vi "数据查询_数据查询.vi"() -> ()   [LabVIEW 2016, in "数据查询.lvlib"]
uses:
  <vilib>/Utility/miscctls.llb/LVPointTypeDef.ctl
  <userlib>/_LVST/sqlite_api/Core/Select/SQLite_Select Str.vi
  <userlib>/_OpenG.lib/array/array.llb/Sort 2D Array (String)__ogtk.vi
  <vilib>/ptbypt/NI_PtbyPt.lvlib
  System.Windows.Forms
panel:
  in  "数据类型":string(combo)="N"
  out "columns":string[](array[string])
  out "表格":string[][](table)
  in  "是否剔除异常数据":bool=TRUE
  in  "WebBrowser":refnum<k24>(container)
  in  "列表框":i32(listbox)
  in  "导出":bool
  in  "测量模式":string(combo)="全部数据"
  out "选中数据表":string
  in  "查询":bool
  in  "结束日期":string="2050/01/01"
  in  "起始日期":string="2010/01/01"
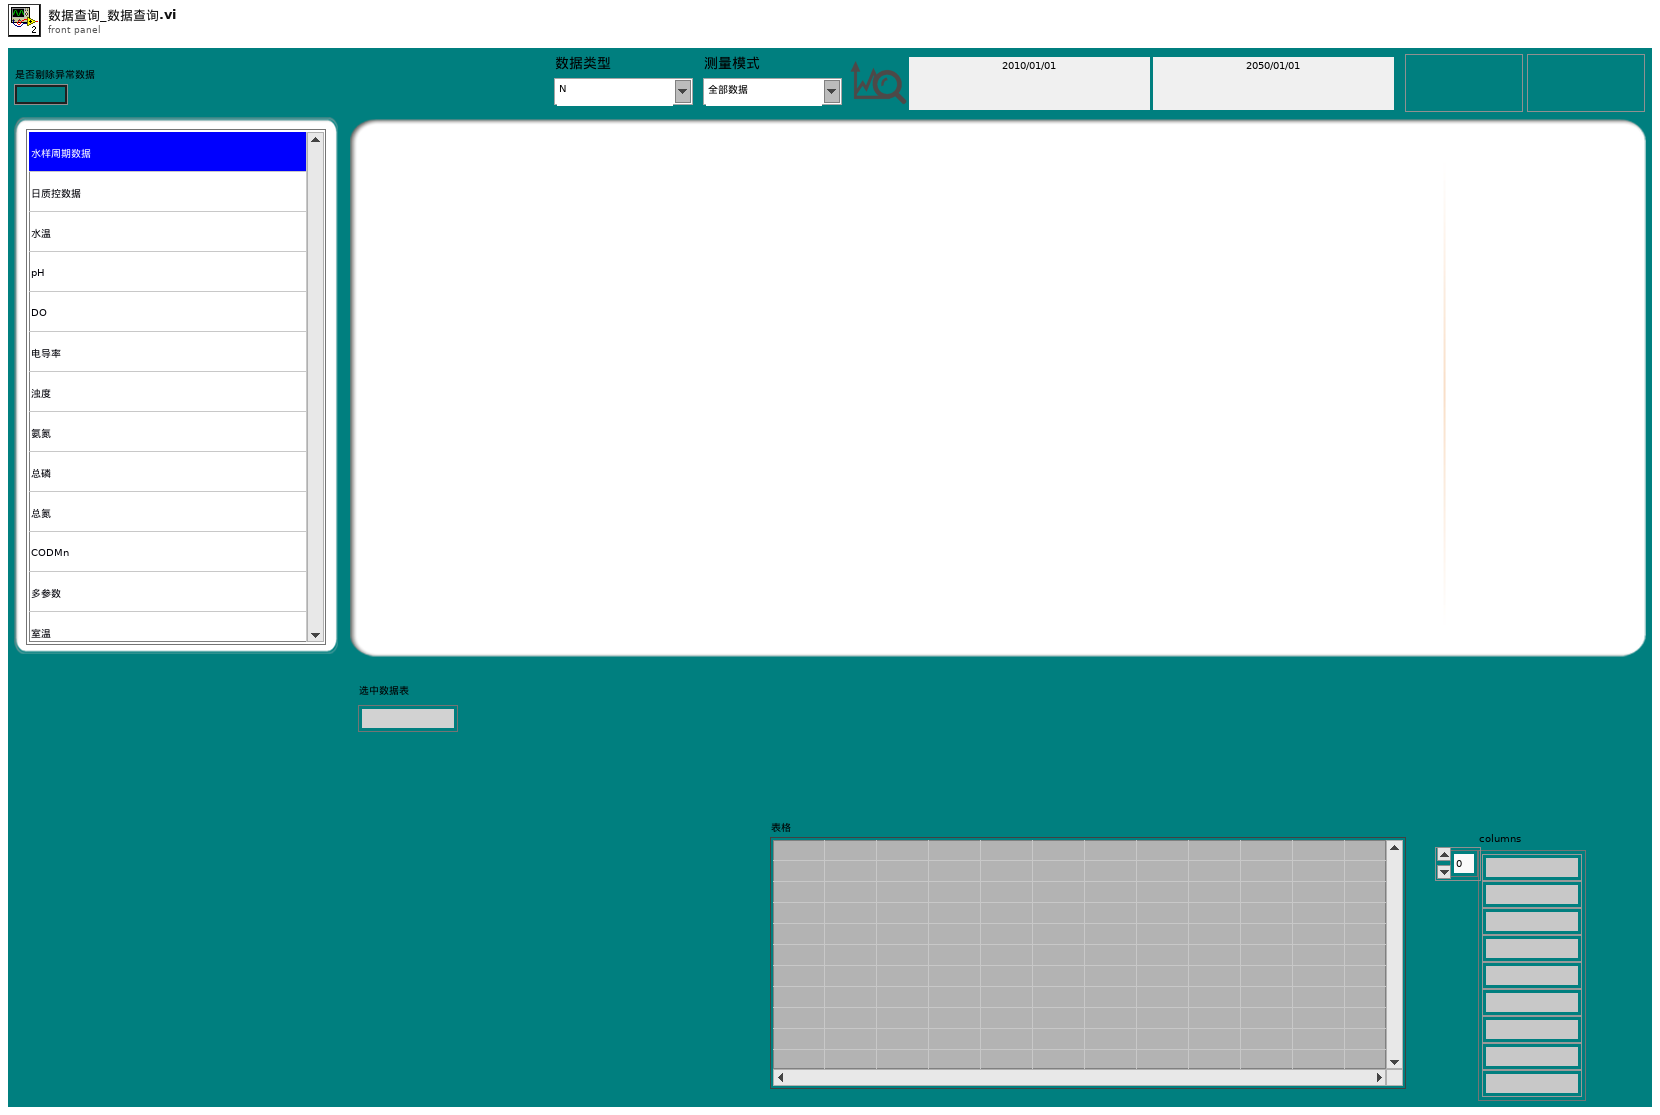
[diagram p1: front panel]
types:
  T1 = typedef "LVPointTypeDef.ctl" = cluster{"Horizontal":i16, "Vertical":i16}
  T2 = typedef "LVDateTimeRec.ctl" = cluster{"秒数的小数部分":dbl, "秒":i32, "分":i32, "时":i32, "日":i32, "月":i32, "年":i32, "天数（周）":i32, "天数（年）":i32, "DST":i32}
  T3 = typedef "数据查询菜单.xctl/数据 1.ctl" = enum32{"数据查询", "仪器数据", "仪器日志", "报警信息", "校准日志"}
  T4 = enum8{"Enabled", "Disabled", "Disabled and Grayed Out"}
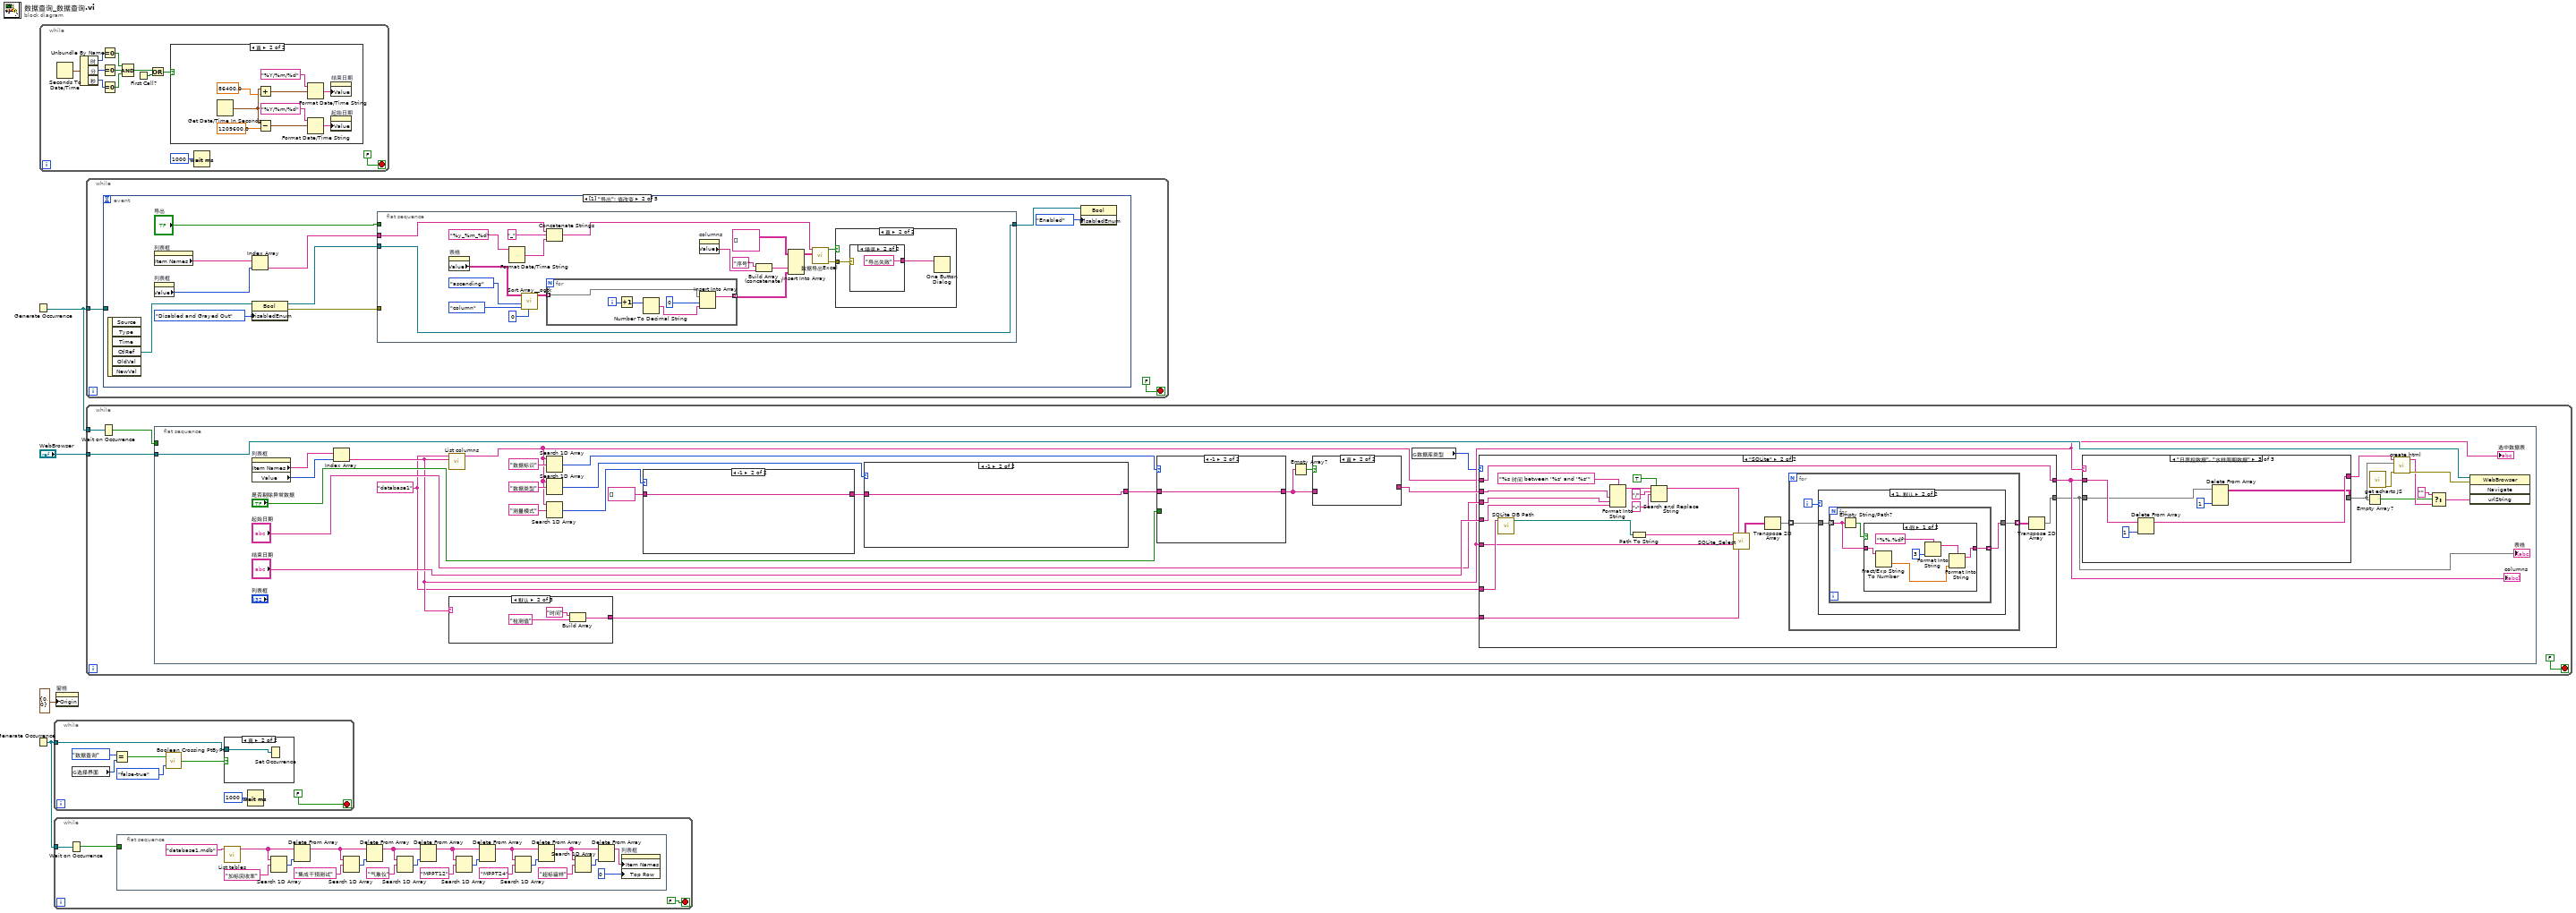
[diagram p0: block diagram]
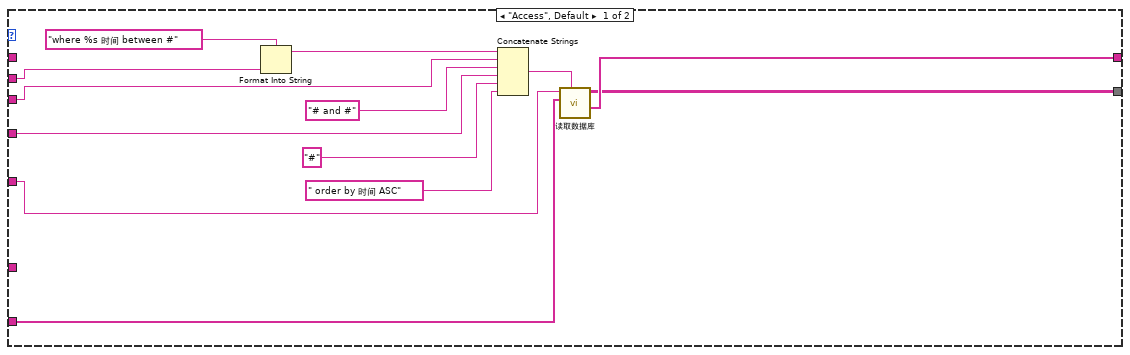
[diagram p3: hidden frame]
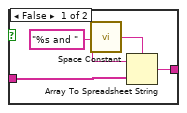
[diagram p6: hidden frame]
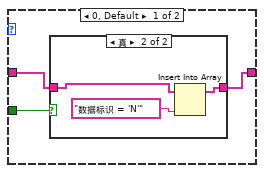
[diagram p7: hidden frame]
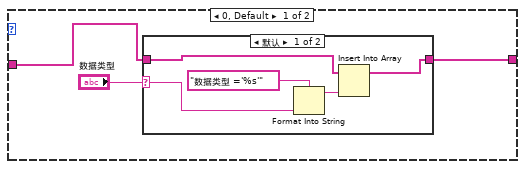
[diagram p9: hidden frame]
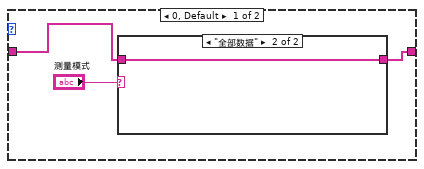
[diagram p11: hidden frame]
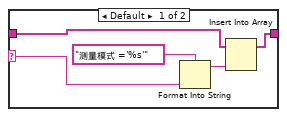
[diagram p12: hidden frame]
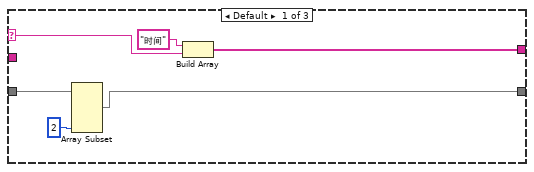
[diagram p13: hidden frame]
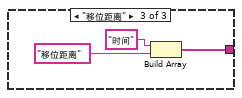
[diagram p16: hidden frame]
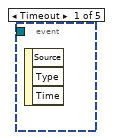
[diagram p18: hidden frame]
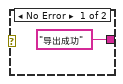
[diagram p20: hidden frame]
diagram:
  n1 = Generate Occurrence() -> (w3:refnum<k4>)
  n2 = Generate Occurrence() -> (w1:refnum<k4>)
  n3 = while {
    stop <- FALSE stop-if-true
    n4 = Seconds To Date/Time() -> (date time rec=w16:T2)  [unwired: 2 in]
    n5 = Unbundle By Name(w16) -> ("时"=w15:i32, "分"=w14:i32, "秒"=w13:i32)
    n6 = Equal To 0?(x=w15) -> (x = 0?=w12:bool)
    n7 = Equal To 0?(x=w14) -> (x = 0?=w11:bool)
    n8 = Equal To 0?(x=w13) -> (x = 0?=w10:bool)
    n9 = Compound Arithmetic op=AND ("复合运算")(w12, w11, w10) -> (w7:bool)
    n10 = First Call?() -> (First Call?: T/F=w5:bool)
    n11 = Or(x=w7, y=w5) -> (x .or. y?=w6:bool)
    n12 = case shown="真" w6 {
      frame False {
      }
      frame True {
        n13 = Get Date/Time In Seconds() -> (seconds since 1Jan1904=w21:timestamp)
        n14 = Add(x=w21, y=86400.0) -> (x+y=w19:timestamp)
        n15 = Subtract(x=w21, y=1209600.0) -> (x-y=w22:timestamp)
        n16 = Format Date/Time String(time format string (%c)="%Y/%m/%d" ("时间格式字符串(%c)"), seconds (now)=w19) -> (date/time string=w18:string)  [unwired: 1 in]
        n17 = Format Date/Time String(time format string (%c)="%Y/%m/%d" ("时间格式字符串(%c)"), seconds (now)=w22) -> (date/time string=w24:string)  [unwired: 1 in]
        n18 = property on="结束日期" class="Str"("Value"=w18) -> ()  [unwired: 2 in, 2 out]
        n19 = property on="起始日期" class="Str"("Value"=w24) -> ()  [unwired: 2 in, 2 out]
      }
    }
    n20 = Wait (ms)(milliseconds to wait=u32 1000 ("等待时间（毫秒）")) -> ()  [unwired: 1 out]
  }
  n21 = while {
    tunnel: w1 -> [w31]
    stop <- FALSE stop-if-true
    n22 = global read "全局变量.vi" "选择界面"() -> (w30:T3)
    n23 = Equal?(x=数据_1."数据查询", y=w30) -> (x = y?=w28:bool)
    n24 = call <vilib>:"Boolean Crossing PtByPt.vi"("direction"=enum16{"either", "false-true", "true-false"}."false-true", "input"=w28) -> ("crossing"=w26:bool)  [unwired: 1 in]
    n25 = case shown="真" w26 {
      tunnel: w31 -> [_ w34]
      frame False {
      }
      frame True {
        n26 = Set Occurrence(w34) -> ()
      }
    }
    n27 = Wait (ms)(milliseconds to wait=u32 1000 ("等待时间（毫秒）")) -> ()  [unwired: 1 out]
  }
  n28 = while {
    tunnel: w1 -> [w36]
    stop <- FALSE stop-if-true
    n29 = Wait on Occurrence(2:w36) -> (0:w35:bool)  [unwired: 2 in]
    n30 = flat-sequence {
      tunnel: w35 -> [_]
      frame #0 {
        n31 = call "List tables.vi"("database"="database1.mdb") -> ("tables"=w42:string[])  [unwired: 9 in, 1 out]
        n32 = Search 1D Array(1D array=w42, element="加标回收率" ("元素")) -> (index of element=w43:i32)  [unwired: 1 in]
        n33 = Delete From Array(array=w42, index=w43) -> (array with subset deleted=w45:string[])  [unwired: 1 in, 1 out]
        n34 = Search 1D Array(1D array=w45, element="集成干预测试" ("元素")) -> (index of element=w44:i32)  [unwired: 1 in]
        n35 = Delete From Array(array=w45, index=w44) -> (array with subset deleted=w48:string[])  [unwired: 1 in, 1 out]
        n36 = Search 1D Array(1D array=w48, element="气象仪" ("元素")) -> (index of element=w46:i32)  [unwired: 1 in]
        n37 = Delete From Array(array=w48, index=w46) -> (array with subset deleted=w51:string[])  [unwired: 1 in, 1 out]
        n38 = Search 1D Array(1D array=w51, element="MPPT12" ("元素")) -> (index of element=w50:i32)  [unwired: 1 in]
        n39 = Delete From Array(array=w51, index=w50) -> (array with subset deleted=w54:string[])  [unwired: 1 in, 1 out]
        n40 = Search 1D Array(1D array=w54, element="MPPT24" ("元素")) -> (index of element=w52:i32)  [unwired: 1 in]
        n41 = Delete From Array(array=w54, index=w52) -> (array with subset deleted=w55:string[])  [unwired: 1 in, 1 out]
        n42 = Search 1D Array(1D array=w55, element="超标留样" ("元素")) -> (index of element=w57:i32)  [unwired: 1 in]
        n43 = Delete From Array(array=w55, index=w57) -> (array with subset deleted=w58:string[])  [unwired: 1 in, 1 out]
        n44 = property on="列表框" class="LstBox (严格)"("Item Names"=w58, "Top Row"=0 ("顶行")) -> ()  [unwired: 2 in, 2 out]
      }
    }
  }
  n45 = property on="窗格" class="Pane"("Origin"=T1 {"Horizontal"=0, "Vertical"=0} ("原点")) -> ()  [unwired: 2 in, 2 out]
  n46 = while {
    tunnel: w3 -> [w59]
    stop <- FALSE stop-if-true
    n47 = event shown="[1] \"导出\": 值改变" {
      selector: _ -> [_ _ _ _ _]
      dyn-events: _ -> [_ _ _ _ _]
      timeout: _ -> [_ _ _ _ _]
      tunnel: w59 -> [_ _ _ w104 w105]
      event Timeout {
        n48 = event-data() -> ()  [unwired: 1 in, 3 out]
      }
      event "导出": Value Change {
        n49 = event-data() -> ("CtlRef"=w70:refnum<vi>)  [unwired: 1 in, 5 out]
        n50 = property on="列表框" class="LstBox (严格)"() -> ("Item Names"=w63:string[])  [unwired: 2 in, 2 out]
        n51 = property on="列表框" class="LstBox (严格)"() -> ("Value"=w62:i32)  [unwired: 2 in, 2 out]
        n52 = Index Array(array=w63, index=w62) -> (element=w61:string)
        n53 = property class="Bool"(reference=w70, "DisabledEnum"=T4."Disabled and Grayed Out" ("禁用")) -> (reference out=w67:refnum<vi>, error out=w68:errorcluster)  [unwired: 1 in]
        n54 = flat-sequence {
          tunnel: w68 -> [_]
          tunnel: [w86] -> w66
          tunnel: w67 -> [w86]
          tunnel: "导出" -> [_]
          tunnel: w61 -> [w76]
          frame #0 {
            n55 = property on="表格" class="Tbl (严格)"() -> ("Value"=w72:string[][])  [unwired: 2 in, 2 out]
            n56 = Format Date/Time String(time format string (%c)="%y_%m_%d" ("时间格式字符串(%c)")) -> (date/time string=w83:string)  [unwired: 2 in]
            n57 = call-poly <userlib>:"Sort Array__ogtk.vi"("Column/Row to Sort By"=u32 0, "Sort By in"=enum16{"row", "column"}."column", "Order"=enum16{"ascending", "descending"}."ascending", "Array in"=w72) -> ("Sorted Array out"=w80:string[][])  [unwired: 4 in, 3 out]
            n58 = Concatenate Strings(w76, "_" ("字符串"), w83) -> (w81:string)
            n59 = for {
              tunnel: w80 -> [w98] mode=indexing
              tunnel: [w97] -> w73 mode=indexing
              i -> [w99]
              n60 = Increment(x=w99) -> (x+1=w95:i32)
              n61 = Number To Decimal String(number=w95) -> (decimal integer string=w94:string)  [unwired: 1 in]
              n62 = Insert Into Array(array=w98, index=0 ("索引"), new element=w94) -> (w97:string[])
            }
            n63 = property on="columns" class="Arr (严格)"() -> ("Value"=w71:string[])  [unwired: 2 in, 2 out]
            n64 = Build Array (concatenate)("序号" ("新元素/子数组"), w71) -> (w74:string[])
            n65 = Insert Into Array(array=string[][] [], new element #1=w74, new element #2=w73) -> (w79:string[][])  [unwired: 2 in]
            n66 = call "数据导出Excel.vi"("text data"=w79, "default name"=w81) -> ("error out"=w78:errorcluster, "布尔"=w77:bool)  [unwired: 8 in]
            n67 = case shown="真" w77 {
              tunnel: w78 -> [_ w91]
              frame False {
              }
              frame True {
                n68 = case shown="错误" w91 {
                  tunnel: ["导出成功" ("消息") "导出失败" ("消息")] -> w90
                  frame No Error {
                  }
                  frame Error {
                  }
                }
                n69 = One Button Dialog(message=w90) -> ()  [unwired: 1 in, 1 out]
              }
            }
          }
        }
        n70 = property class="Bool"(reference=w66, "DisabledEnum"=T4."Enabled" ("禁用")) -> ()  [unwired: 1 in, 2 out]
      }
      event "起始日期", "结束日期": Mouse Down {
        n71 = event-data() -> ("CtlRef"=w103:refnum<vi>)  [unwired: 1 in, 7 out]
        n72 = property class="Str"(reference=w103) -> (reference out=w101:refnum<vi>, "Value"=w102:string)  [unwired: 1 in, 1 out]
        n73 = call "日期键盘.vi"("原值"=w102) -> ("x+y"=w100:string)  [unwired: 10 in]
        n74 = property class="Str"(reference=w101, "Val(Sgnl)"=w100) -> ()  [unwired: 1 in, 2 out]
      }
      event "查询", "起始日期", "结束日期", "测量模式", "是否剔除异常数据", "数据类型": Value Change {
        n75 = event-data() -> ()  [unwired: 1 in, 6 out]
        n76 = Set Occurrence(w104) -> ()
      }
      event "列表框": Value Change; "列表框": Mouse Down {
        n77 = event-data() -> ()  [unwired: 1 in, 4 out]
        n78 = flat-sequence {
          tunnel: [w107] -> w106
          tunnel: w105 -> [w107]
          tunnel: w106 -> [w110]
          frame #0 {
            n79 = property on="测量模式" class="CmbBox"("Value"="全部数据" ("测量模式")) -> ()  [unwired: 2 in, 2 out]
            n80 = property on="数据类型" class="CmbBox"("Value"="N" ("数据类型")) -> ()  [unwired: 2 in, 2 out]
          }
          frame #1 {
            n81 = Set Occurrence(w110) -> ()
          }
        }
      }
    }
  }
  n82 = while {
    tunnel: w3 -> [w113]
    tunnel: "WebBrowser" -> [w111]
    stop <- FALSE stop-if-true
    n83 = Wait on Occurrence(2:w113) -> (0:w112:bool)  [unwired: 2 in]
    n84 = flat-sequence {
      tunnel: w112 -> [_]
      tunnel: w111 -> [w145]
      frame #0 {
        w115 = "database1" ("database")
        n85 = property on="列表框" class="LstBox (严格)"() -> ("Item Names"=w137:string[], "Value"=w136:i32)  [unwired: 2 in, 2 out]
        n86 = Index Array(array=w137, index=w136) -> (element=w128:string)
        "选中数据表" <- w128
        n87 = call "List columns.vi"("table"=w128, "database"=w115) -> ("columns"=w116:string[])  [unwired: 8 in, 1 out]
        n88 = case shown="默认" w128 {
          tunnel: [_ w242 w245] -> w139
          frame "多参数", "环境参数", "日质控数据", "水样周期数据" {
          }
          frame Default {
            n89 = Build Array("时间", "检测值") -> (w242:string[])
          }
          frame "移位距离" {
            n90 = Build Array("时间", "移位距离") -> (w245:string[])
          }
        }
        n91 = Search 1D Array(1D array=w116, element="数据标识" ("元素")) -> (index of element=w120:i32)  [unwired: 1 in]
        n92 = Search 1D Array(1D array=w116, element="数据类型" ("元素")) -> (index of element=w121:i32)  [unwired: 1 in]
        n93 = Search 1D Array(1D array=w116, element="测量模式" ("元素")) -> (index of element=w123:i32)  [unwired: 1 in]
        n94 = case shown="-1" w123 {
          tunnel: string[] [] -> [w220 w227]
          tunnel: [w218 w227] -> w122
          frame 0, Default {
            n95 = case shown="\"全部数据\"" "测量模式" {
              selector: "测量模式" -> [w224 _]
              tunnel: w220 -> [w223 w226]
              tunnel: [w221 w226] -> w218
              frame Default {
                n96 = Format Into String(format string="测量模式 ='%s'" ("condition"), w224) -> (resulting string=w222:string)  [unwired: 2 in, 1 out]
                n97 = Insert Into Array(array=w223, new element=w222) -> (w221:string[])  [unwired: 1 in]
              }
              frame "全部数据" {
              }
            }
          }
          frame -1 {
          }
        }
        n98 = case shown="-1" w121 {
          tunnel: [w209 w217] -> w124
          tunnel: w122 -> [w208 w217]
          frame 0, Default {
            n99 = case shown="默认" "数据类型" {
              selector: "数据类型" -> [w214 _]
              tunnel: w208 -> [w213 w216]
              tunnel: [w211 w216] -> w209
              frame Default {
                n100 = Format Into String(format string="数据类型 ='%s'" ("condition"), w214) -> (resulting string=w212:string)  [unwired: 2 in, 1 out]
                n101 = Insert Into Array(array=w213, new element=w212) -> (w211:string[])  [unwired: 1 in]
              }
              frame "全部数据" {
              }
            }
          }
          frame -1 {
          }
        }
        n102 = case shown="-1" w120 {
          tunnel: "是否剔除异常数据" -> [w202 _]
          tunnel: [w201 w207] -> w119
          tunnel: w124 -> [w200 w207]
          frame 0, Default {
            n103 = case shown="真" w202 {
              tunnel: w200 -> [w203 w206]
              tunnel: [w203 w204] -> w201
              frame False {
              }
              frame True {
                n104 = Insert Into Array(array=w206, new element="数据标识 = 'N'" ("condition")) -> (w204:string[])  [unwired: 1 in]
              }
            }
          }
          frame -1 {
          }
        }
        n105 = Empty Array?(array=w119) -> (empty?=w118:bool)
        n106 = case shown="真" w118 {
          tunnel: [w199 _] -> w129
          tunnel: w119 -> [w196 _]
          frame False {
            n107 = call <vilib>:"Space Constant.vi"() -> ("String"=w198:string)
            n108 = Array To Spreadsheet String(delimiter (Tab)=w198, array=w196, 3:"%s and " ("格式字符串")) -> (spreadsheet string=w199:string)
          }
          frame True {
          }
        }
        n109 = global read "全局变量.vi" "数据库类型"() -> (w117:enum16{"Access", "SQLite"})
        n110 = case shown="\"SQLite\"" w117 {
          tunnel: "结束日期" -> [w156 w166]
          tunnel: "起始日期" -> [w155 w167]
          tunnel: [w154 w164] -> w142
          tunnel: [w153 w165] -> w140
          tunnel: w139 -> [w152 w162]
          tunnel: w129 -> [w151 w168]
          tunnel: w128 -> [w148 w161]
          tunnel: w116 -> [_ w164]
          tunnel: w115 -> [_ w163]
          frame "Access", Default {
            n111 = Format Into String(format string="where %s 时间 between #" ("condition"), w151) -> (resulting string=w149:string)  [unwired: 2 in, 1 out]
            n112 = Concatenate Strings(w149, w155, "# and #" ("condition"), w156, "#" ("condition"), " order by 时间 ASC" ("字符串")) -> (w160:string)
            n113 = call "读取数据库.vi"("condition"=w160, "显示项"=w152, "组合框"=w148) -> ("columns"=w154:string[], "表格"=w153:string[][])  [unwired: 5 in, 2 out]
          }
          frame "SQLite" {
            n114 = call "SQLite DB Path.vi"("database"=w163) -> ("appended path"=w179:path)  [unwired: 10 in]
            n115 = Format Into String(format string="%s 时间 between '%s' and '%s'" ("格式字符串"), w168, w167, w166) -> (resulting string=w173:string)  [unwired: 2 in, 1 out]
            n116 = Path To String(path=w179) -> (string=w178:string)
            n117 = Search and Replace String(replace all?=TRUE ("替换全部？(F)"), input string=w173, search string="/" ("搜索字符串"), replace string="-" ("替换字符串(\"\")")) -> (result string=w172:string)  [unwired: 4 in, 3 out]
            n118 = call-poly <userlib>:"SQLite_Select.vi"("DB Path"=w178, "Where Clause"=w172, "Table Name"=w161, "Columns"=w162) -> ("Results"=w171:string[][])  [unwired: 8 in, 3 out]
            n119 = Transpose 2D Array(2D array=w171) -> (transposed array=w170:string[][])
            n120 = for {
              tunnel: w170 -> [w182] mode=indexing
              tunnel: [w181] -> w169 mode=indexing
              i -> [w180]
              n121 = case shown="1, 默认" w180 {
                tunnel: w182 -> [w183 w185]
                tunnel: [w183 w184] -> w181
                frame 0 {
                }
                frame 1, Default {
                  n122 = for {
                    tunnel: w185 -> [w187] mode=indexing
                    tunnel: [w188] -> w184 mode=indexing
                    n123 = Empty String/Path?(string/path=w187) -> (empty?=w186:bool)
                    n124 = case shown="假" w186 {
                      tunnel: [w192 w195] -> w188
                      tunnel: w187 -> [w189 w195]
                      frame False {
                        n125 = Fract/Exp String To Number(string=w189) -> (number=w191:dbl)  [unwired: 3 in, 1 out]
                        n126 = Format Into String(format string="%%.%df" ("格式字符串"), 3 ("输入 1")) -> (resulting string=w194:string)  [unwired: 2 in, 1 out]
                        n127 = Format Into String(format string=w194, w191) -> (resulting string=w192:string)  [unwired: 2 in, 1 out]
                      }
                      frame True {
                      }
                    }
                  }
                }
              }
            }
            n128 = Transpose 2D Array(2D array=w169) -> (transposed array=w165:string[][])
          }
        }
        "表格" <- w140
        "columns" <- w142
        n129 = case shown="\"日质控数据\", \"水样周期数据\"" w128 {
          selector: w128 -> [w230 _ _]
          tunnel: w142 -> [_ w235 w241]
          tunnel: [w229 w235 w240] -> w141
          tunnel: w140 -> [w233 w234 w238]
          tunnel: [w232 w234 w237] -> w132
          frame Default {
            n130 = Array Subset(array=w233, length (col)=2 ("长度")) -> (w232:string[][])  [unwired: 3 in]
            n131 = Build Array("时间", w230) -> (w229:string[])
          }
          frame "多参数", "环境参数" {
          }
          frame "日质控数据", "水样周期数据" {
            n132 = Delete From Array(array=w241, index=1 ("索引")) -> (array with subset deleted=w240:string[])  [unwired: 1 in, 1 out]
            n133 = Delete From Array(array=w238, index (col)=1 ("禁用的索引 (列)")) -> (array with subset deleted=w237:string[][])  [unwired: 2 in, 1 out]
          }
        }
        n134 = Empty Array?(array=w132) -> (empty?=w131:bool)
        n135 = call "get echarts JS.vi"() -> ("error out"=w144:errorcluster)  [unwired: 11 in]
        n136 = call "create html.vi"("error in (no error)"=w144, "data"=w132, "columns"=w141) -> ("error out"=w143:errorcluster, "url"=w135:string)  [unwired: 7 in]
        n137 = Select(t="", s=w131, f=w135) -> (s? t:f=w134:string)
        n138 = invoke class="WebBrowser" method="Navigate"(reference=w145, error in=w143, "urlString"=w134) -> ()  [unwired: 1 in, 4 out]
      }
    }
  }
